vi "SOUR_POW_STOP.vi"(0 "VISA IN":refnum<visa-resource-name>, 1 "Stop Power":dbl, 5 "error in":errorcluster, 7 "Channel":i32) -> (14 "VISA Out":refnum<visa-resource-name>, 19 "error out":errorcluster)   [LabVIEW 2018, in "PNA-X.lvlib"]
doc: "SOURce<cnum>:POWer:STOP <num> \n1832\n\n(Read-Write) Sets the power sweep stop power. Must also set: SENS:SWE:TYPE POWer and \nSOURce:POWer:START <num>. \nParameters \n<cnum> Any existing channel number. If unspecified, value is set to 1 \n<num> Stop power. \nNote: The range of settable power values depends on the PNA model and if \nsource attenuators are installed. To determine the range of values, perform a \nquery using MAX, then MIN, as an argument. (SOUR:POW:ATT:AUTO must \nbe set to ON) Example: SOURce:POWer:STOP? MAX \nActual achievable leveled power depends on frequency. \nExamples SOUR:POW:STOP -15 \nsource2:power:stop -7 \nQuery Syntax SOURce<cnum>:POWer:STOP? \nReturn Type Numeric \nDefault 0 dBm \nLast modified: \n10/18/06 MQQ Added Mode command \n1833\n\nSource:Power:Correction Commands \nControls the source power calibration features of the analyzer. \nClick on a blue keyword to view the command details. \nSee Also \nExample program using these commands. \nTemplate for creating your own Power Meter Driver \nLearn about Source Power Cal \nSynchronizing the PNA and Controller \nSCPI Command Tree \nNote: The SOURce:POWer:CORRection:COLLect:ACQuire command, used to step the PNA and read a \npower meter, cannot be sent over the GPIB unless the power meter is connected to a different GPIB \ninterface. See the alternative methods described in the command details."
uses:
  PNA-X.lvlib
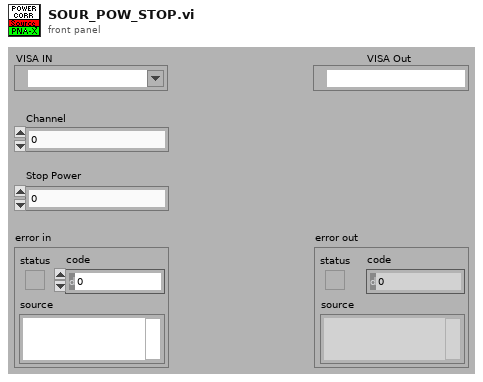
[diagram p1: front panel]
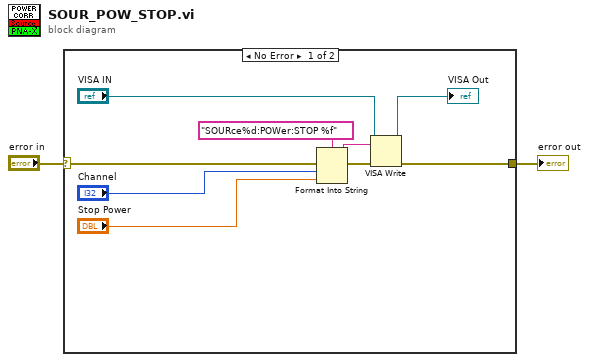
[diagram p0: block diagram]
diagram:
  n1 = case shown="No Error" "error in" {
    selector: "error in" -> [w11 w12]
    tunnel: [w9 w12] -> w1
    frame No Error {
      n2 = Format Into String(format string="SOURce%d:POWer:STOP %f" ("Cmdline"), error in=w11, "Channel", "Stop Power") -> (resulting string=w4:string, error out=w5:errorcluster)  [unwired: 1 in]
      n3 = VISA Write(VISA resource name="VISA IN", write buffer=w4, error in (no error)=w5) -> (VISA resource name out=→"VISA Out":refnum<visa-resource-name>, error out=w9:errorcluster)  [unwired: 1 out]
    }
    frame Error {
    }
  }
  "error out" <- w1
